vi "Station.Execution.vi"() -> ()   [LabVIEW 2015, in "Station.Execution.lvlib"]
uses:
  Station.Execution.lvlib
  Types/Main.StateVariables.ctl
  Types/Execute.UserEventRefs.ctl
  <vilib>/NI Veristand/Execution/Workspace/SystemStateRegEventRef.ctl
  <vilib>/NI Veristand/Execution/Workspace/Target State Info.ctl
  <vilib>/NI Veristand/Execution/Workspace/Target State.ctl
  <vilib>/NI Veristand/Execution/WaveformStreaming/Waveform Data Watcher Event Data (DBL).ctl
  <vilib>/NI Veristand/Execution/WaveformStreaming/WaveformStreamSpecification.ctl
  <vilib>/NI Veristand/Execution/Workspace/SystemStateEventRef.ctl
  <vilib>/NI Veristand/Execution/Workspace/WorkspaceAPI.ctl
  Types/UI.Tables.ctl
  Types/UI.Object.ctl
  Types/Waveforms.Info.ctl
  <vilib>/NI Veristand/Execution/WaveformStreaming/Registered Waveform Streams Data Event Refnum (DBL).ctl
  <vilib>/NI Veristand/Execution/WaveformStreaming/WaveformDataWatcherDBL.ctl
  <vilib>/NI Veristand/Execution/WaveformStreaming/WaveformStreamingAPI.ctl
  <vilib>/NI/AMC/Read Termination Message.vi
  <vilib>/NI/AMC/Update Message Routing Info.vi
  <vilib>/NI/AMC/Create Multiple Messages.vi
  <vilib>/NI/AMC/Create Single Message.vi
  <vilib>/NI/AMC/Globals.vi
  <vilib>/NI/AMC/Send Message.vi
  NationalInstruments.VeriStand.ClientAPI
  <vilib>/NI Veristand/Execution/Workspace/NI_VS Workspace ExecutionAPI.lvlib
  <vilib>/NI/AMC/AMC.lvlib
  <vilib>/NI Veristand/Execution/WaveformStreaming/NI_VS Waveform Streaming Interface.lvlib
panel:
  in  "Station.ID":string="DUT1"
  out "Station ID":string="Station 1"
  in  "NIVS.Gateway IP Address":string="localhost"
  in  "NIVS.Workspace Event":refnum<event-registration>
  in  "ToolTab":enum32{"Enable", "Disable"}(tab)
  in  "Back":bool
  in  "Next":bool
  in  "Pages":T1(tab)
  out "CAN.ODH":string[][](table)
  out "DAQ.ODH":string[][](table)
  out "CAN.IDL":string[][](table)
  out "DAQ.IDL":string[][](table)
  out "CAN.IDH":string[][](table)
  out "DAQ.IDH":string[][](table)
  out "CAN.OPH":string[][](table)
  out "DAQ.OPH":string[][](table)
  out "CAN.ODL":string[][](table)
  out "DAQ.ODL":string[][](table)
  out "CAN.Fault Status":string[][](table)
  out "CAN.LIN":string[][](table)
  in  "Waveform.Select":bool
  out "Waveform.Graph":waveform(dbl)[](graph)
  in  "Waveform.Groups":u8(ring) items=["", "All", "Eat", "Slow", "Test"]
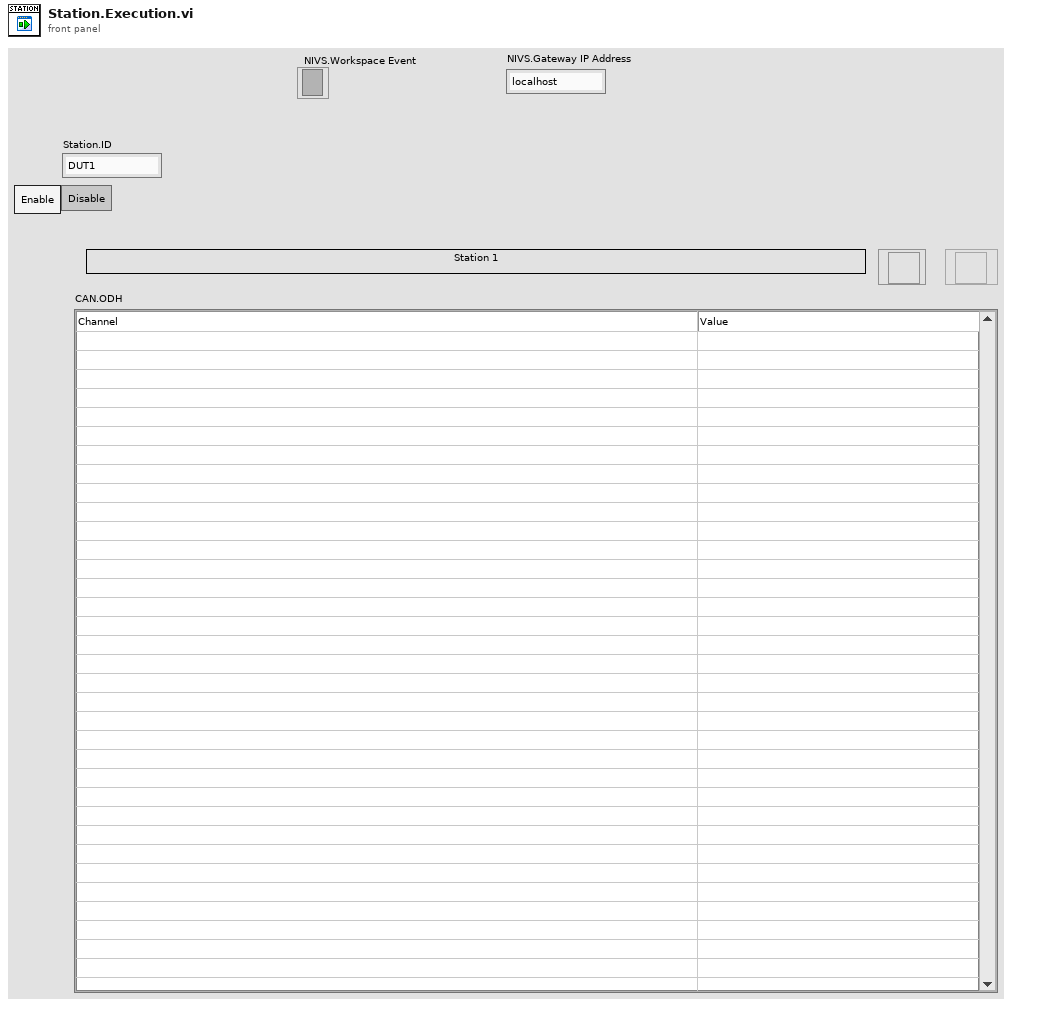
[diagram p1: front panel]
types:
  T1 = enum32{"CAN.ODH", "DAQ.ODH", "CAN.IDL", "DAQ.IDL", "CAN.IDH", "DAQ.IDH", "CAN.OPH", "DAQ.OPH", "CAN.ODL", "DAQ.ODL", "CAN.Fault Status", "CAN.LIN", "OSCOPE"}
  T2 = typedef "Station.Execution.lvlib/Main.StateVariables.ctl" = cluster{"NIVS.Deployed":bool, "NIVS.Events":T3, "NIVS.GatewayIPAddress":string, "NIVS.SystemDefinitionFile":path, "NIVS.SystemStateRefs":T5, "NIVS.WorkspaceManager":T6, "Station.ID":string, "UI.Back":refnum<vi>, "UI.Next":refnum<vi>, "UI.Pages":refnum<vi>, "UI.ToolTab":refnum<vi>, "Tables":T7, "VI.Ref":refnum<vi>, "NIVS.Open":bool, "Waveform.Groups":refnum<vi>, "Waveform.Select":refnum<vi>, "Waveform.Graph":refnum<vi>, "Waveforms.Info":T9[], "Waveforms":cluster{"Refs":T10[], "Event.Refs":T11, "Streaming.Ref":T13}, "Waveforms.Reset":bool}
  T3 = typedef "Station.Execution.lvlib/Execute.UserEventRefs.ctl" = cluster{"SystemChangeEvent":T4, "WorkspaceEvent":refnum<event-registration>, "WaveformEvent":refnum<event-registration>}
  T4 = typedef "NI_VS Workspace ExecutionAPI.lvlib/SystemStateRegEventRef.ctl" = refnum<event-registration>
  T5 = typedef "NI_VS Workspace ExecutionAPI.lvlib/SystemStateEventRef.ctl" = cluster{"CustDatRef":refnum<user-event>, "EvtRef":refnum<k27>, "Target State User Event":refnum<user-event>}
  T6 = typedef "NI_VS Workspace ExecutionAPI.lvlib/WorkspaceAPI.ctl" = refnum<k24>
  T7 = typedef "Station.Execution.lvlib/UI.Tables.ctl" = cluster{"CAN.Fault Status":T8, "CAN.IDH":T8, "CAN.IDL":T8, "CAN.LIN":T8, "CAN.ODH":T8, "CAN.ODL":T8, "CAN.OPH":T8, "DAQ.IDH":T8, "DAQ.IDL":T8, "DAQ.ODH":T8, "DAQ.ODL":T8, "DAQ.OPH":T8}
  T8 = typedef "Station.Execution.lvlib/UI.Object.ctl" = cluster{"Ref":refnum<vi>, "Paths":string[], "Names":string[]}
  T9 = typedef "Station.Execution.lvlib/Waveforms.Info.ctl" = cluster{"Name":string, "Path":string}
  T10 = typedef "NI_VS Waveform Streaming Interface.lvlib/WaveformStreamSpecification.ctl" = refnum<k24>
  T11 = typedef "NI_VS Waveform Streaming Interface.lvlib/Registered Waveform Streams Data Event Refnum (DBL).ctl" = cluster{"Callback Refnum":refnum<k27>, "Data Event":refnum<user-event>, "Event Refnum":refnum<event-registration>, "WaveformDataWatcherDBL":T12}
  T12 = typedef "NI_VS Waveform Streaming Interface.lvlib/WaveformDataWatcherDBL.ctl" = refnum<k24>
  T13 = typedef "NI_VS Waveform Streaming Interface.lvlib/WaveformStreamingAPI.ctl" = refnum<k24>
  T14 = typedef "AMC.lvlib/Message Queue.ctl" = refnum<queue>
  T15 = enum8{"Enabled", "Disabled", "Disabled and Grayed Out"}
  T16 = cluster{"Waveform.Refs":T10[], "WaveformStreaming.Event.Refs":T11, "WaveformStreaming.Ref":T13}
  T17 = typedef "AMC.lvlib/Message.ctl" = cluster{"name":string, "value":string, "attributes":T18, "receiver host":string, "receiver process":string, "source host":string, "source process":string, "priority message":bool, "acknowledge message":bool}
  T18 = typedef "Tools_KeyedArray.lvlib/KeyedArray.ctl" = cluster{"keys":string[], "values":string[]}
  T19 = cluster{"Refs":T10[], "Event.Refs":T11, "Streaming.Ref":T13}
  T20 = typedef "NI_VS Workspace ExecutionAPI.lvlib/SystemState.ctl" = u8
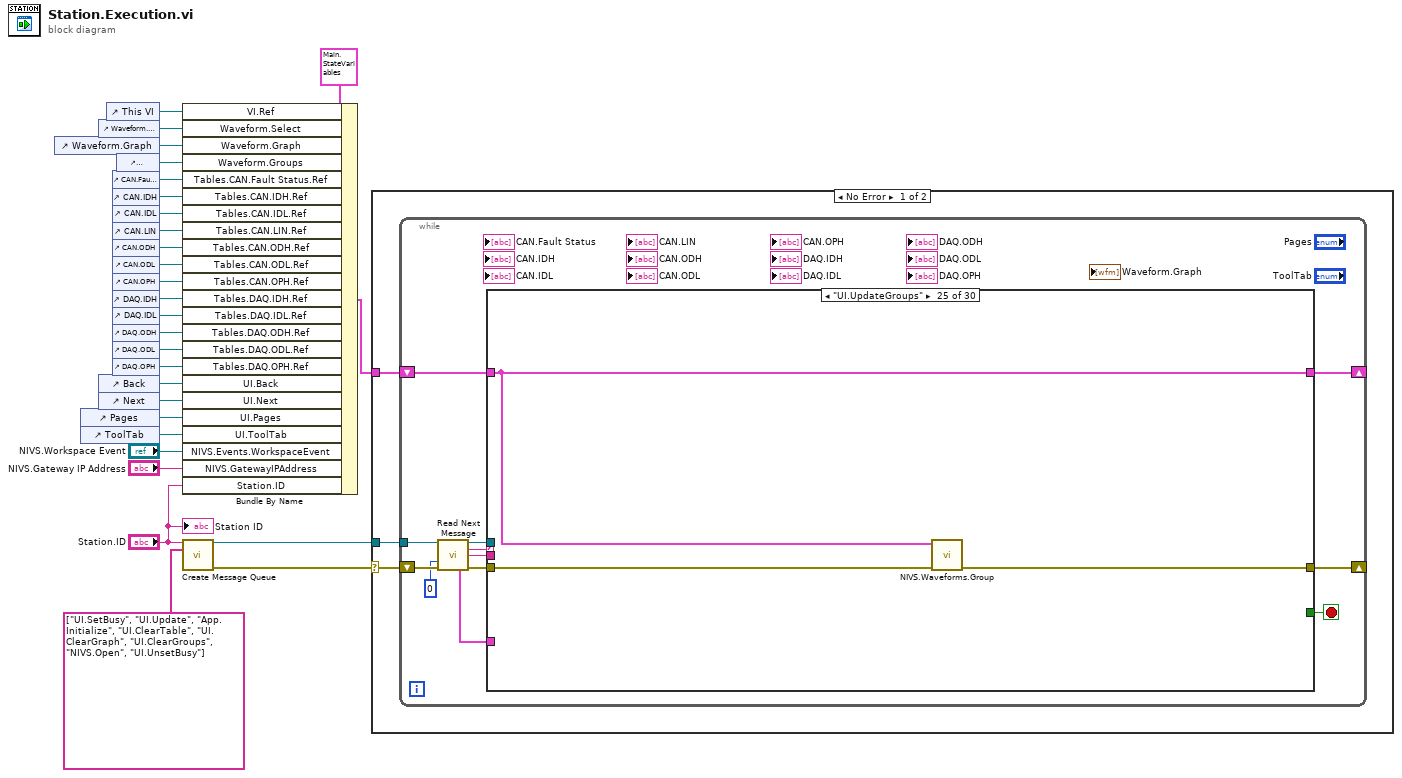
[diagram p0: block diagram]
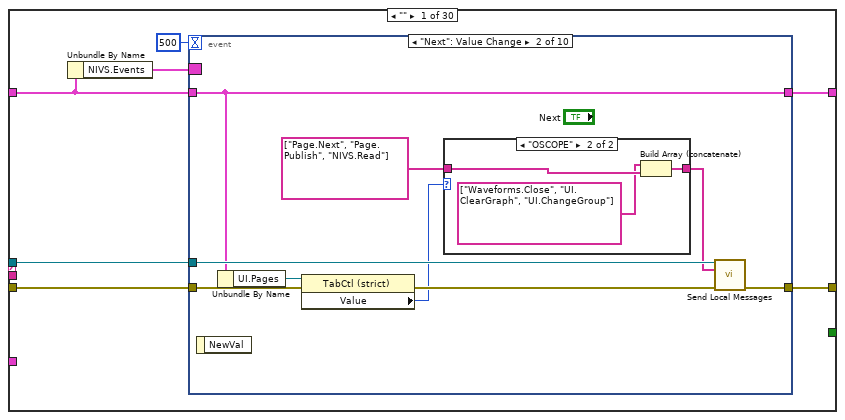
[diagram p2: hidden frame]
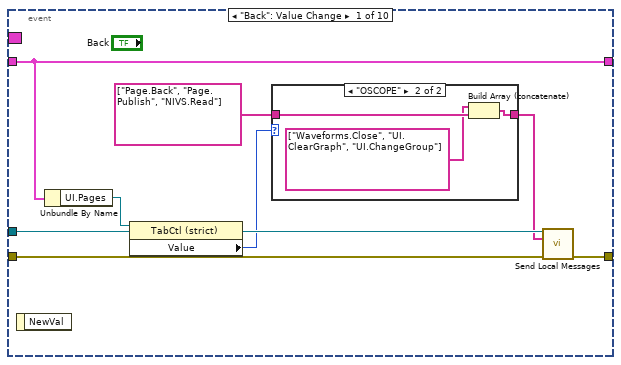
[diagram p3: hidden frame]
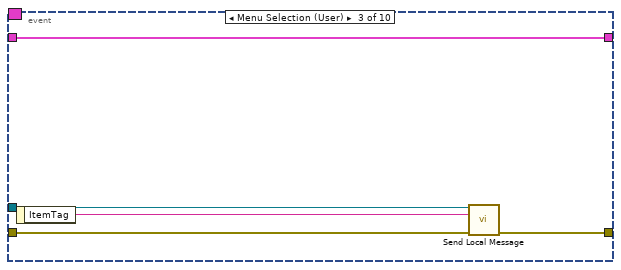
[diagram p6: hidden frame]
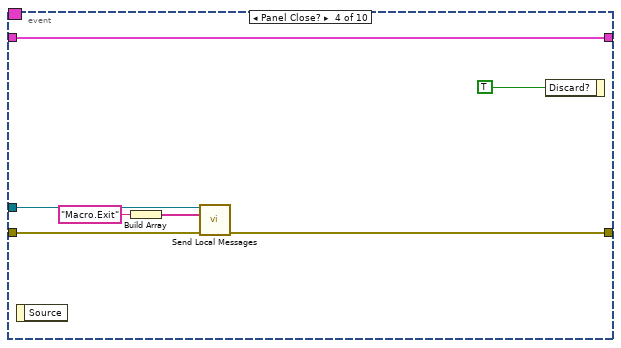
[diagram p7: hidden frame]
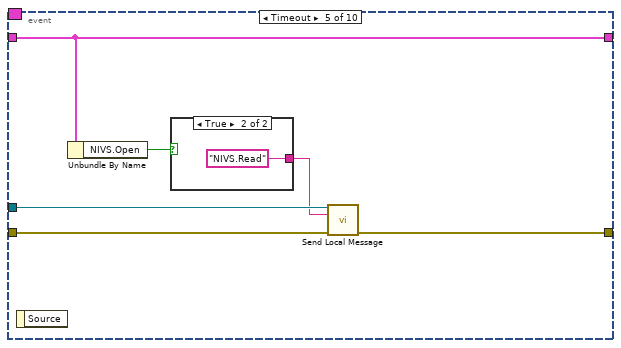
[diagram p8: hidden frame]
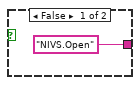
[diagram p9: hidden frame]
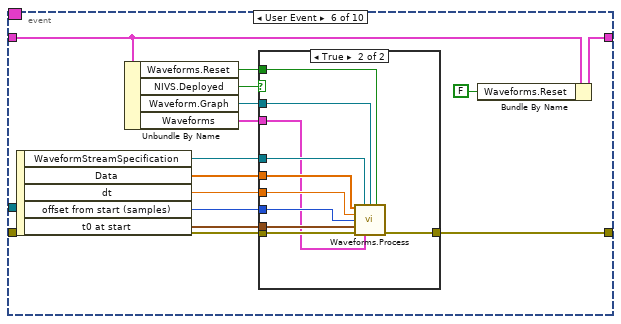
[diagram p10: hidden frame]
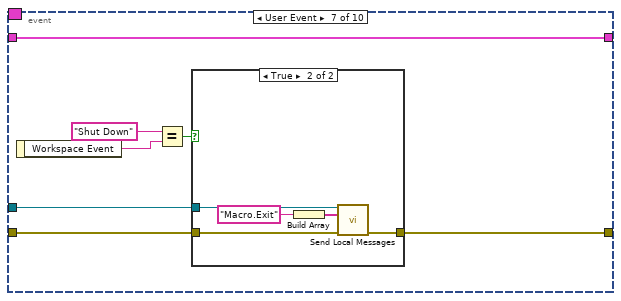
[diagram p12: hidden frame]
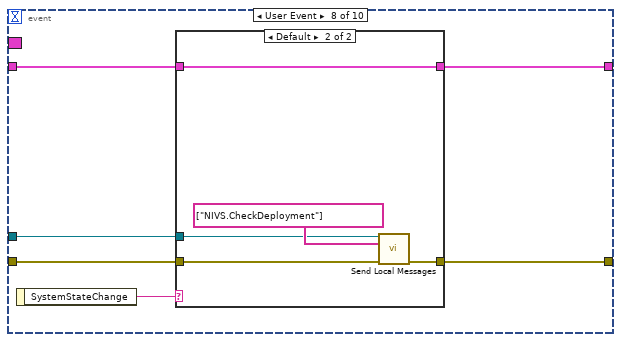
[diagram p14: hidden frame]
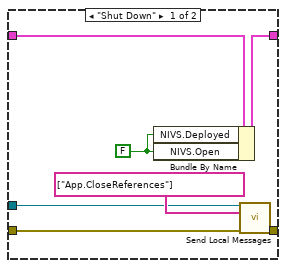
[diagram p15: hidden frame]
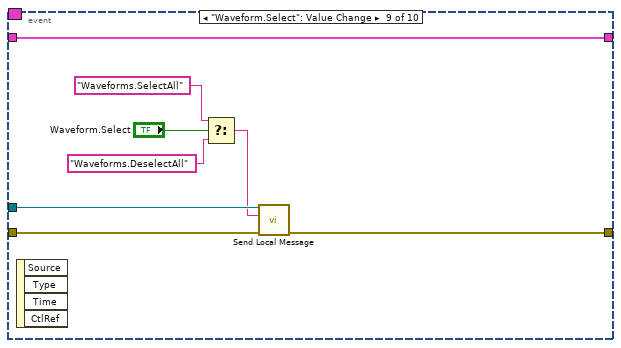
[diagram p16: hidden frame]
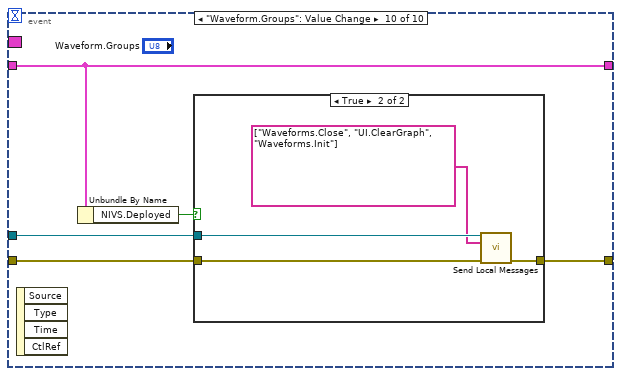
[diagram p17: hidden frame]
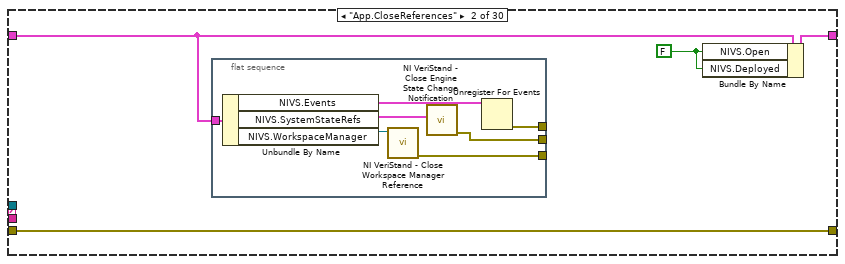
[diagram p19: hidden frame]
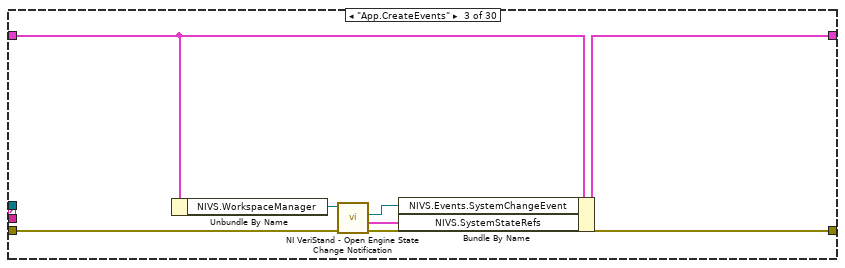
[diagram p20: hidden frame]
diagram:
  n1 = control-ref of="Waveform.Graph"() -> (w1:refnum<vi>)
  n2 = control-ref of="Pages"() -> (w5:refnum<vi>)
  n3 = control-ref of="ToolTab"() -> (w23:refnum<vi>)
  n4 = control-ref of="Waveform.Select"() -> (w2:refnum<vi>)
  n5 = control-ref of="Back"() -> (w21:refnum<vi>)
  n6 = control-ref of="Next"() -> (w22:refnum<vi>)
  n7 = control-ref of="This VI"() -> (w4:refnum<vi>)
  n8 = control-ref of="CAN.Fault Status"() -> (w16:refnum<vi>)
  n9 = control-ref of="CAN.IDH"() -> (w15:refnum<vi>)
  n10 = control-ref of="CAN.IDL"() -> (w14:refnum<vi>)
  n11 = control-ref of="CAN.LIN"() -> (w13:refnum<vi>)
  n12 = control-ref of="CAN.ODH"() -> (w12:refnum<vi>)
  n13 = control-ref of="CAN.ODL"() -> (w11:refnum<vi>)
  n14 = control-ref of="CAN.OPH"() -> (w10:refnum<vi>)
  n15 = control-ref of="DAQ.IDH"() -> (w9:refnum<vi>)
  n16 = control-ref of="DAQ.IDL"() -> (w8:refnum<vi>)
  n17 = control-ref of="DAQ.ODH"() -> (w17:refnum<vi>)
  n18 = control-ref of="DAQ.ODL"() -> (w18:refnum<vi>)
  n19 = control-ref of="DAQ.OPH"() -> (w19:refnum<vi>)
  n20 = control-ref of="Waveform.Groups"() -> (w3:refnum<vi>)
  n21 = Bundle By Name(cluster=T2 {"NIVS.Deployed"=FALSE, "NIVS.Events"={"SystemChangeEvent"=refnum, "WorkspaceEvent"=refnum, "WaveformEvent"=refnum}, "NIVS.GatewayIPAddress"="", "NIVS.SystemDefinitionFile"=path "", "NIVS.SystemStateRefs"={"CustDatRef"=refnum, "EvtRef"=refnum, "Target State User Event"=refnum}, "NIVS.WorkspaceManager"=refnum, "Station.ID"="", "UI.Back"=refnum, "UI.Next"=refnum, "UI.Pages"=refnum, "UI.ToolTab"=refnum, "Tables"={"CAN.Fault Status"={"Ref"=refnum, "Paths"=[], "Names"=[]}, "CAN.IDH"={"Ref"=refnum, "Paths"=[], "Names"=[]}, "CAN.IDL"={"Ref"=refnum, "Paths"=[], "Names"=[]}, "CAN.LIN"={"Ref"=refnum, "Paths"=[], "Names"=[]}, "CAN.ODH"={"Ref"=refnum, "Paths"=[], "Names"=[]}, "CAN.ODL"={"Ref"=refnum, "Paths"=[], "Names"=[]}, "CAN.OPH"={"Ref"=refnum, "Paths"=[], "Names"=[]}, "DAQ.IDH"={"Ref"=refnum, "Paths"=[], "Names"=[]}, "DAQ.IDL"={"Ref"=refnum, "Paths"=[], "Names"=[]}, "DAQ.ODH"={"Ref"=refnum, "Paths"=[], "Names"=[]}, "DAQ.ODL"={"Ref"=refnum, "Paths"=[], "Names"=[]}, "DAQ.OPH"={"Ref"=refnum, "Paths"=[], "Names"=[]}}, "VI.Ref"=refnum, "NIVS.Open"=FALSE, "Waveform.Groups"=refnum, "Waveform.Select"=refnum, "Waveform.Graph"=refnum, "Waveforms.Info"=[], "Waveforms"={"Refs"=[], "Event.Refs"={"Callback Refnum"=refnum, "Data Event"=refnum, "Event Refnum"=refnum, "WaveformDataWatcherDBL"=refnum}, "Streaming.Ref"=refnum}, "Waveforms.Reset"=FALSE} ("Cluster"), "VI.Ref"=w4, "Waveform.Select"=w2, "Waveform.Graph"=w1, "Waveform.Groups"=w3, "Tables.CAN.Fault Status.Ref"=w16, "Tables.CAN.IDH.Ref"=w15, "Tables.CAN.IDL.Ref"=w14, "Tables.CAN.LIN.Ref"=w13, "Tables.CAN.ODH.Ref"=w12, "Tables.CAN.ODL.Ref"=w11, "Tables.CAN.OPH.Ref"=w10, "Tables.DAQ.IDH.Ref"=w9, "Tables.DAQ.IDL.Ref"=w8, "Tables.DAQ.ODH.Ref"=w17, "Tables.DAQ.ODL.Ref"=w18, "Tables.DAQ.OPH.Ref"=w19, "UI.Back"=w21, "UI.Next"=w22, "UI.Pages"=w5, "UI.ToolTab"=w23, "NIVS.Events.WorkspaceEvent"="NIVS.Workspace Event", "NIVS.GatewayIPAddress"="NIVS.Gateway IP Address", "Station.ID"="Station.ID") -> (w28:T2)
  n22 = call <vilib>:"Create Message Queue.vi"("message queue name"="Station.ID", "initial message names"=string[] ["UI.SetBusy", "UI.Update", "App.Initialize", "UI.ClearTable", "UI.ClearGraph", "UI.ClearGroups", "NIVS.Open", "UI.UnsetBusy"]) -> ("message queue out"=w25:T14, "error out"=w6:errorcluster)  [unwired: 12 in]
  n23 = case shown="No Error" w6 {
    selector: w6 -> [w29 _]
    tunnel: w28 -> [w30 _]
    tunnel: w25 -> [w31 _]
    frame No Error {
      n24 = while {
        shift-right: [w42] -> _
        shift-left: w30 -> [w43]
        shift-right: [w32] -> _
        shift-left: w29 -> [w41]
        tunnel: w31 -> [w39]
        stop <- w40 stop-if-true
        n25 = call <vilib>:"Read Next Message.vi"("message queue in"=w39, "timeout (1 ms)"=0 ("Timeout"), "error in"=w41) -> ("message queue out"=w36:T14, "message name"=w35:string, "message value"=w34:string, "message"=w33:T17, "error out"=w37:errorcluster)  [unwired: 5 in, 3 out]
        n26 = case shown="\"UI.UpdateGroups\"" w35 {
          selector: w35 -> [_ _ _ _ _ _ _ _ _ _ _ _ _ _ _ _ _ w338 w344 _ _ _ _ _ _ _ _ _ _ _]
          tunnel: w43 -> [w46 w172 w181 w188 w193 w199 w214 w218 w237 w267 w271 w272 w293 w324 w328 w331 w333 w342 w347 w355 w358 w370 w376 w381 w384 w387 w396 w412 w436 w447]
          tunnel: [w50 w171 w182 w188 w193 w199 w214 w217 w236 w263 w271 w272 w293 w324 w328 w331 w332 w342 w347 w355 w358 w370 w376 w381 w384 w386 w395 w412 w436 w447] -> w42
          tunnel: [w47 w173 w184 w189 w194 w203 w212 w224 w238 w265 w269 w274 w292 w310 w325 w329 w334 w339 w343 w348 w356 w368 w373 w378 w382 w385 w397 w401 w425 w446] -> w32
          tunnel: w37 -> [w48 w173 w183 w190 w195 w202 w213 w219 w239 w268 w270 w273 w291 w310 w326 w330 w334 w339 w343 w349 w357 w363 w374 w379 w383 w390 w394 w404 w428 w446]
          tunnel: [_ _ _ TRUE _ _ _ _ _ _ _ _ _ _ _ _ _ _ _ _ _ _ _ _ _ _ _ _ _ _] -> w40
          tunnel: w36 -> [w44 _ _ w191 _ w200 w211 w223 w235 _ _ _ _ _ _ _ _ _ _ _ _ _ _ _ _ _ _ _ _ _]
          tunnel: w34 -> [_ _ _ _ _ _ _ _ _ _ _ _ _ _ w327 _ _ _ _ _ _ _ _ _ _ _ _ _ _ _]
          tunnel: w33 -> [_ _ _ _ _ _ _ _ _ _ _ _ _ _ _ _ _ _ _ _ _ _ _ _ _ _ _ _ _ _]
          frame "" {
            n27 = Unbundle By Name(w46) -> ("NIVS.Events"=w45:T3)
            n28 = event shown="[1] \"Next\": Value Change" {
              selector: w45 -> [_ _ _ _ _ _ _ _ _ _]
              dyn-events: _ -> [_ _ _ _ _ _ _ _ _ _]
              timeout: 500 -> [_ _ _ _ _ _ _ _ _ _]
              tunnel: [w52 w69 w76 w86 w89 w97 w125 w134 w159 w161] -> w50
              tunnel: w46 -> [w52 w69 w76 w86 w89 w98 w125 w135 w159 w161]
              tunnel: [w57 w71 w79 w83 w91 w108 w123 w136 w157 w163] -> w47
              tunnel: w48 -> [w58 w67 w80 w84 w92 w109 w124 w139 w158 w164]
              tunnel: w44 -> [w56 w70 w78 w82 w93 _ w122 w138 w156 w162]
              event "Back": Value Change {
                n29 = event-data() -> ()  [unwired: 1 in, 1 out]
                n30 = Unbundle By Name(w52) -> ("UI.Pages"=w51:refnum<vi>)
                n31 = property class="TabCtl (strict)"(reference=w51) -> ("Value"=w55:T1)  [unwired: 1 in, 2 out]
                n32 = case shown="\"OSCOPE\"" w55 {
                  tunnel: [w59 w61] -> w54
                  tunnel: string[] ["Page.Back", "Page.Publish", "NIVS.Read"] ("message names") -> [w59 w62]
                  frame Default {
                  }
                  frame "OSCOPE" {
                    n33 = Build Array (concatenate)(string[] ["Waveforms.Close", "UI.ClearGraph", "UI.ChangeGroup"], w62) -> (w61:string[])
                  }
                }
                n34 = call <vilib>:"Send Local Messages.vi"("message queue in"=w56, "message names"=w54, "error in"=w58) -> ("error out"=w57:errorcluster)  [unwired: 10 in, 2 out]
              }
              event "Next": Value Change {
                n35 = event-data() -> ()  [unwired: 1 in, 1 out]
                n36 = Unbundle By Name(w69) -> ("UI.Pages"=w68:refnum<vi>)
                n37 = property class="TabCtl (strict)"(reference=w68, error in=w67) -> (error out=w66:errorcluster, "Value"=w65:T1)  [unwired: 1 out]
                n38 = case shown="\"OSCOPE\"" w65 {
                  tunnel: [w72 w74] -> w63
                  tunnel: string[] ["Page.Next", "Page.Publish", "NIVS.Read"] ("message names") -> [w72 w75]
                  frame Default {
                  }
                  frame "OSCOPE" {
                    n39 = Build Array (concatenate)(string[] ["Waveforms.Close", "UI.ClearGraph", "UI.ChangeGroup"], w75) -> (w74:string[])
                  }
                }
                n40 = call <vilib>:"Send Local Messages.vi"("message queue in"=w70, "message names"=w63, "error in"=w66) -> ("error out"=w71:errorcluster)  [unwired: 10 in, 2 out]
              }
              event Menu Selection (User) {
                n41 = event-data() -> ("ItemTag"=w77:string)  [unwired: 1 in]
                n42 = call <vilib>:"Send Local Message.vi"("message queue in"=w78, "message name"=w77, "error in"=w80) -> ("error out"=w79:errorcluster)  [unwired: 10 in, 2 out]
              }
              event Panel Close? {
                n43 = event-data() -> ()  [unwired: 1 in, 1 out]
                n44 = Build Array("Macro.Exit") -> (w81:string[])
                n45 = call <vilib>:"Send Local Messages.vi"("message queue in"=w82, "message names"=w81, "error in"=w84) -> ("error out"=w83:errorcluster)  [unwired: 10 in, 2 out]
                n46 = event-data("Discard?"=TRUE) -> ()  [unwired: 1 in, 1 out]
              }
              event Timeout {
                n47 = event-data() -> ()  [unwired: 1 in, 1 out]
                n48 = Unbundle By Name(w89) -> ("NIVS.Open"=w88:bool)
                n49 = case shown="True" w88 {
                  tunnel: ["NIVS.Open" ("message name") "NIVS.Read" ("message name")] -> w90
                  frame False {
                  }
                  frame True {
                  }
                }
                n50 = call <vilib>:"Send Local Message.vi"("message queue in"=w93, "message name"=w90, "error in"=w92) -> ("error out"=w91:errorcluster)  [unwired: 10 in, 2 out]
              }
              event User Event {
                n51 = event-data() -> ("WaveformStreamSpecification"=w107:T10, "Data"=w105:dbl[], "dt"=w104:dbl, "offset from start (samples)"=w103:u64, "t0 at start"=w102:timestamp)  [unwired: 1 in]
                n52 = Unbundle By Name(w98) -> ("Waveforms.Reset"=w99:bool, "NIVS.Deployed"=w100:bool, "Waveform.Graph"=w106:refnum<vi>, "Waveforms"=w101:T19)
                n53 = case shown="True" w100 {
                  tunnel: w109 -> [w110 w120]
                  tunnel: [w110 w119] -> w108
                  tunnel: w107 -> [_ w118]
                  tunnel: w106 -> [_ w117]
                  tunnel: w105 -> [_ w116]
                  tunnel: w104 -> [_ w115]
                  tunnel: w103 -> [_ w114]
                  tunnel: w102 -> [_ w113]
                  tunnel: w101 -> [_ w112]
                  tunnel: w99 -> [_ w111]
                  frame False {
                  }
                  frame True {
                    n54 = call "Waveforms.Process.vi"("Data"=w116, "Waveform.Ref"=w118, "WaveformGraph.Ref"=w117, "Reset?"=w111, "dt"=w115, "offset from start (samples)"=w114, "t0 at start"=w113, "error in (no error)"=w120, "Waveforms"=w112) -> ("error out"=w119:errorcluster)  [unwired: 6 in]
                  }
                }
                n55 = Bundle By Name(cluster=w98, "Waveforms.Reset"=FALSE) -> (w97:T2)
              }
              event User Event {
                n56 = event-data() -> ("Workspace Event"=w121:string)  [unwired: 1 in]
                n57 = Equal?(x="Shut Down" ("y"), y=w121) -> (x = y?=w126:bool)
                n58 = case shown="True" w126 {
                  tunnel: w124 -> [w128 w133]
                  tunnel: [w128 w132] -> w123
                  tunnel: w122 -> [_ w131]
                  frame False {
                  }
                  frame True {
                    n59 = Build Array("Macro.Exit" ("y")) -> (w130:string[])
                    n60 = call <vilib>:"Send Local Messages.vi"("message queue in"=w131, "message names"=w130, "error in"=w133) -> ("error out"=w132:errorcluster)  [unwired: 10 in, 2 out]
                  }
                }
              }
              event User Event {
                n61 = event-data() -> ("SystemStateChange"=w137:string)  [unwired: 1 in]
                n62 = case shown="Default" w137 {
                  tunnel: w139 -> [w145 w150]
                  tunnel: w138 -> [w144 w149]
                  tunnel: [w143 w148] -> w136
                  tunnel: w135 -> [w142 w147]
                  tunnel: [w141 w147] -> w134
                  frame "Shut Down" {
                    w140 = FALSE ("NIVS.Open")
                    n63 = Bundle By Name(cluster=w142, "NIVS.Deployed"=w140, "NIVS.Open"=w140) -> (w141:T2)
                    n64 = call <vilib>:"Send Local Messages.vi"("message queue in"=w144, "message names"=string[] ["App.CloseReferences"], "error in"=w145) -> ("error out"=w143:errorcluster)  [unwired: 10 in, 2 out]
                  }
                  frame Default {
                    n65 = call <vilib>:"Send Local Messages.vi"("message queue in"=w149, "message names"=string[] ["NIVS.CheckDeployment"], "error in"=w150) -> ("error out"=w148:errorcluster)  [unwired: 10 in, 2 out]
                  }
                }
              }
              event "Waveform.Select": Value Change {
                n66 = event-data() -> ()  [unwired: 1 in, 4 out]
                n67 = Select(t="Waveforms.SelectAll", s="Waveform.Select", f="Waveforms.DeselectAll") -> (s? t:f=w152:string)
                n68 = call <vilib>:"Send Local Message.vi"("message queue in"=w156, "message name"=w152, "error in"=w158) -> ("error out"=w157:errorcluster)  [unwired: 10 in, 2 out]
              }
              event "Waveform.Groups": Value Change {
                n69 = event-data() -> ()  [unwired: 1 in, 4 out]
                n70 = Unbundle By Name(w161) -> ("NIVS.Deployed"=w160:bool)
                n71 = case shown="True" w160 {
                  tunnel: w164 -> [w165 w169]
                  tunnel: [w165 w168] -> w163
                  tunnel: w162 -> [_ w167]
                  frame False {
                  }
                  frame True {
                    n72 = call <vilib>:"Send Local Messages.vi"("message queue in"=w167, "message names"=string[] ["Waveforms.Close", "UI.ClearGraph", "Waveforms.Init"], "error in"=w169) -> ("error out"=w168:errorcluster)  [unwired: 10 in, 2 out]
                  }
                }
              }
            }
          }
          frame "App.CloseReferences" {
            w170 = FALSE ("NIVS.Open")
            n73 = flat-sequence {
              tunnel: w172 -> [w177]
              tunnel: [w176] -> _
              tunnel: [w175] -> _
              tunnel: [w174] -> _
              frame #0 {
                n74 = Unbundle By Name(w177) -> ("NIVS.Events"=w178:T3, "NIVS.SystemStateRefs"=w180:T5, "NIVS.WorkspaceManager"=w179:T6)
                n75 = call <vilib>:"NI VeriStand - Close Workspace Manager Reference.vi"("WorkspaceManager"=w179) -> ("error out"=w174:errorcluster)  [unwired: 10 in]
                n76 = call <vilib>:"NI VeriStand - Close Engine State Change Notification.vi"("SystemStateRefs"=w180) -> ("error out"=w175:errorcluster)  [unwired: 10 in]
                n77 = Unregister For Events(event registration refnum=w178) -> (error out=w176:errorcluster)  [unwired: 1 in]
              }
            }
            n78 = Bundle By Name(cluster=w172, "NIVS.Open"=w170, "NIVS.Deployed"=w170) -> (w171:T2)
          }
          frame "App.CreateEvents" {
            n79 = Unbundle By Name(w181) -> ("NIVS.WorkspaceManager"=w185:T6)
            n80 = call <vilib>:"NI VeriStand - Open Engine State Change Notification.vi"("error in (no error)"=w183, "WorkspaceManager in"=w185) -> ("error out"=w184:errorcluster, "SystemStateRefs"=w187:T5, "SystemChangeEventRef"=w186:T4)  [unwired: 6 in, 1 out]
            n81 = Bundle By Name(cluster=w181, "NIVS.Events.SystemChangeEvent"=w186, "NIVS.SystemStateRefs"=w187) -> (w182:T2)
          }
          frame "App.Exit" {
            n82 = call <vilib>:"Destroy Message Queue.vi"("message queue in"=w191, "error in"=w190) -> ("error out"=w189:errorcluster)  [unwired: 11 in, 2 out]
          }
          frame "App.Initialize" {
            n83 = call "Execute.Initialize.vi"("error in (no error)"=w195, "State Variables"=w193) -> ("error out"=w194:errorcluster)  [unwired: 9 in]
          }
          frame "Error" {
            n84 = for {
              shift-right: [w208] -> w197
              shift-left: w202 -> [w209]
              tunnel: i32[] [-307652, -307654] -> [w207] mode=indexing
              n85 = call <vilib>:"Clear Errors.vi"("error in (no error)"=w209, "specific error code to clear (0: all)"=w207) -> ("error out"=w208:errorcluster)  [unwired: 4 in, 1 out]
            }
            n86 = case shown="Error" w197 {
              selector: w197 -> [w204 w205]
              tunnel: [w204 w206] -> w198
              frame No Error {
              }
              frame Error {
                n87 = call <vilib>:"Clear Errors.vi"("error in (no error)"=w205) -> ("error out"=w206:errorcluster)  [unwired: 5 in, 1 out]
                n88 = call "Error.Display.vi"("error in (no error)"=w205) -> ()  [unwired: 11 in]
              }
            }
            n89 = call <vilib>:"Send Local Messages.vi"("message queue in"=w200, "message names"=string[] ["UI.SetBusy", "UI.Update", "App.CloseReferences", "App.Initialize", "UI.ClearTable", "NIVS.Open", "UI.UnsetBusy"], "error in"=w198) -> ("error out"=w203:errorcluster)  [unwired: 10 in, 2 out]
          }
          frame "Macro.Exit" {
            n90 = call <vilib>:"Send Local Messages.vi"("message queue in"=w211, "message names"=string[] ["Waveforms.Close", "App.CloseReferences", "UI.Close", "App.Exit"], "error in"=w213) -> ("error out"=w212:errorcluster)  [unwired: 10 in, 2 out]
          }
          frame "NIVS.CheckDeployment" {
            n91 = Unbundle By Name(w218) -> ("NIVS.WorkspaceManager"=w221:T6)
            n92 = call <vilib>:"NI VeriStand - Get System State.vi"("error in (no error)"=w219, "WorkspaceManager in"=w221) -> ("error out"=w215:errorcluster, "System State"=w222:T20, "System Definition File"=w220:path)  [unwired: 5 in, 2 out]
            n93 = case shown="0, Default" w222 {
              tunnel: w218 -> [w229 w234]
              tunnel: [w228 w232] -> w217
              tunnel: w220 -> [_ w231]
              tunnel: [string[] ["Waveforms.Close", "UI.Update", "UI.ClearTable", "UI.ClearGraph", "UI.ClearGroups", "NIVS.GetChannels"] string[] ["UI.Update", "NIVS.GetChannels", "UI.UpdateGroups"]] -> w216
              frame 0, Default {
                # "Not connected"
                n94 = Bundle By Name(cluster=w229, "NIVS.Deployed"=FALSE ("Connected"), "NIVS.SystemDefinitionFile"=path "") -> (w228:T2)
              }
              frame 1 {
                # "Connected"
                n95 = Bundle By Name(cluster=w234, "NIVS.Deployed"=TRUE ("Connected"), "NIVS.SystemDefinitionFile"=w231) -> (w232:T2)
              }
            }
            n96 = call <vilib>:"Send Local Messages.vi"("message queue in"=w223, "message names"=w216, "error in"=w215) -> ("error out"=w224:errorcluster)  [unwired: 10 in, 2 out]
          }
          frame "NIVS.Open" {
            n97 = Unbundle By Name(w237) -> ("NIVS.GatewayIPAddress"=w240:string)
            n98 = case shown="No Error" w239 {
              selector: w239 -> [w243 w261]
              tunnel: w240 -> [w248 _]
              tunnel: [w242 w261] -> w238
              tunnel: w237 -> [w246 w262]
              tunnel: [w244 w262] -> w236
              tunnel: w235 -> [w241 _]
              frame No Error {
                n99 = call <vilib>:"NI VeriStand - Open Workspace Manager Reference.vi"("Gateway IP Address (\"\": localhost)"=w248) -> ("error out"=w247:errorcluster, "WorkspaceManager"=w245:T6)  [unwired: 9 in]
                n100 = case shown="No Error" w247 {
                  tunnel: w246 -> [w256 w259]
                  tunnel: w245 -> [w255 _]
                  tunnel: [w253 w258] -> w244
                  tunnel: w243 -> [w252 w260]
                  tunnel: [w251 w260] -> w242
                  tunnel: w241 -> [w250 _]
                  frame No Error {
                    n101 = Bundle By Name(cluster=w256, "NIVS.Open"=TRUE, "NIVS.WorkspaceManager"=w255) -> (w253:T2)
                    n102 = call <vilib>:"Send Local Messages.vi"("message queue in"=w250, "message names"=string[] ["App.CreateEvents", "NIVS.CheckDeployment"], "error in"=w252) -> ("error out"=w251:errorcluster)  [unwired: 10 in, 2 out]
                  }
                  frame Error {
                    n103 = Bundle By Name(cluster=w259, "NIVS.Open"=FALSE) -> (w258:T2)
                  }
                }
              }
              frame Error {
              }
            }
          }
          frame "NIVS.GetChannels" {
            n104 = call "NIVS.FilterChannels.vi"("error in (no error)"=w268, "Cluster in"=w267) -> ("error out"=w266:errorcluster, "Cluster out"=w264:T2)  [unwired: 8 in]
            n105 = call "NIVS.FilterWaveforms.vi"("error in (no error)"=w266, "Cluster in"=w264) -> ("error out"=w265:errorcluster, "Cluster out"=w263:T2)  [unwired: 8 in]
          }
          frame "NIVS.Read" {
            n106 = call "NIVS.Channels.Read.vi"("error in (no error)"=w270, "State Variables"=w271) -> ("error out"=w269:errorcluster)  [unwired: 9 in]
          }
          frame "Page.Back" {
            n107 = Unbundle By Name(w272) -> ("UI.Next"=w276:refnum<vi>, "UI.Back"=w283:refnum<vi>, "UI.Pages"=w288:refnum<vi>)
            n108 = property class="TabCtl (strict)"(reference=w288, error in=w273) -> (reference out=w286:refnum<vi>, error out=w285:errorcluster, "Value"=w287:T1)
            n109 = Decrement(x=w287) -> (x-1=w282:T1)
            n110 = Equal To 0?(x=w282) -> (x = 0?=w281:bool)
            n111 = property class="TabCtl (strict)"(reference=w286, error in=w285, "Value"=w282) -> (error out=w284:errorcluster)  [unwired: 1 out]
            n112 = Select(t=T15."Disabled and Grayed Out" ("Disabled"), s=w281, f=T15."Enabled") -> (s? t:f=w278:T15)
            n113 = property class="Bool"(reference=w283, error in=w284, "DisabledEnum"=w278) -> (error out=w277:errorcluster)  [unwired: 1 out]
            n114 = property class="Bool"(reference=w276, error in=w277, "DisabledEnum"=T15."Enabled" ("Disabled")) -> (error out=w274:errorcluster)  [unwired: 1 out]
          }
          frame "Page.Next" {
            n115 = Unbundle By Name(w293) -> ("UI.Back"=w309:refnum<vi>, "UI.Next"=w308:refnum<vi>, "UI.Pages"=w307:refnum<vi>)
            n116 = property class="TabCtl (strict)"(reference=w307, error in=w291) -> (reference out=w295:refnum<vi>, error out=w296:errorcluster, "Value"=w294:T1, "Pages"=w290:refnum<vi>[])
            n117 = To Unsigned Byte Integer(number=w294) -> (unsigned 8bit integer=w306:u8)
            n118 = Array Size(array=w290) -> (size(s)=w289:i32)
            n119 = Increment(x=w306) -> (x+1=w297:u8)
            n120 = Increment(x=w297) -> (x+1=w298:u8)
            n121 = property class="TabCtl (strict)"(reference=w295, error in=w296, "Value"=w297) -> (error out=w299:errorcluster)  [unwired: 1 out]
            n122 = Greater Or Equal?(x=w298, y=w289) -> (x >= y?=w304:bool)
            n123 = Select(t=T15."Disabled and Grayed Out" ("Disabled"), s=w304, f=T15."Enabled") -> (s? t:f=w305:T15)
            n124 = property class="Bool"(reference=w308, error in=w299, "DisabledEnum"=w305) -> (error out=w300:errorcluster)  [unwired: 1 out]
            n125 = property class="Bool"(reference=w309, error in=w300, "DisabledEnum"=T15."Enabled" ("Disabled")) -> (error out=w292:errorcluster)  [unwired: 1 out]
          }
          frame "Page.Publish" {
            n126 = Unbundle By Name(w324) -> ("Station.ID"=w318:string, "UI.Pages"=w323:refnum<vi>)
            n127 = property class="TabCtl (strict)"(reference=w323, error in=w310) -> (error out=w319:errorcluster, "Value"=w321:T1, "Pages"=w322:refnum<vi>[])  [unwired: 1 out]
            n128 = Index Array(array=w322, index=w321) -> (element=w320:refnum<vi>)
            n129 = property class="Page"(reference=w320, error in=w319) -> (error out=w314:errorcluster, "PageLabel"=w317:string)  [unwired: 1 out]
            n130 = Concatenate Strings(w318, "\\" ("string"), w317) -> (w315:string)
            n131 = call <vilib>:"Send Local Message.vi"("receiver process (\"\" - local)"="MainExecutionTool" ("string"), "message name"="Page.Published" ("string"), "message value"=w315, "error in"=w314) -> ("error out"=w311:errorcluster)  [unwired: 9 in, 2 out]
            n132 = call <vilib>:"Clear Errors.vi"("error in (no error)"=w311) -> ()  [unwired: 5 in, 2 out]
          }
          frame "Page.Set" {
            n133 = call "Page.Set.vi"("error in (no error)"=w326, "message value"=w327, "Cluster"=w328) -> ("error out"=w325:errorcluster)  [unwired: 8 in]
          }
          frame "UI.Open" {
            n134 = invoke class="VI" method="FP.Open"(error in=w330) -> (error out=w329:errorcluster)  [unwired: 4 in, 4 out]
          }
          frame "UI.Close" {
            n135 = flat-sequence {
              tunnel: [w336] -> w332
              tunnel: w333 -> [w336]
              tunnel: [w335] -> _
              frame #0 {
                n136 = invoke class="VI" method="FP.Close"() -> (error out=w335:errorcluster)  [unwired: 3 in, 2 out]
                n137 = Wait (ms)(milliseconds to wait=u32 500) -> ()  [unwired: 1 out]
              }
            }
          }
          frame "UI.SetBusy" {
            n138 = call <vilib>:"Send Local Message.vi"("receiver process (\"\" - local)"="MainExecutionTool" ("string"), "message name"=w338, "error in"=w339) -> ("error out"=w340:errorcluster)  [unwired: 10 in, 2 out]
            n139 = call <vilib>:"Clear Errors.vi"("error in (no error)"=w340) -> ()  [unwired: 5 in, 2 out]
            n140 = call <vilib>:"Set Busy.vi"() -> ()  [unwired: 10 in, 2 out]
          }
          frame "UI.UnsetBusy" {
            n141 = call <vilib>:"Send Local Message.vi"("receiver process (\"\" - local)"="MainExecutionTool" ("string"), "message name"=w344, "error in"=w343) -> ("error out"=w345:errorcluster)  [unwired: 10 in, 2 out]
            n142 = call <vilib>:"Clear Errors.vi"("error in (no error)"=w345) -> ()  [unwired: 5 in, 2 out]
            n143 = call <vilib>:"Unset Busy.vi"() -> ()  [unwired: 11 in, 1 out]
          }
          frame "UI.Update" {
            n144 = Unbundle By Name(w355) -> ("UI.ToolTab"=w354:refnum<vi>, "NIVS.Deployed"=w353:bool)
            n145 = Select(t=enum32{"Enable", "Disable"}."Enable" ("Value"), s=w353, f=enum32{"Enable", "Disable"}."Disable") -> (s? t:f=w350:enum32{"Enable", "Disable"})
            n146 = property class="TabCtl (strict)"(reference=w354, error in=w349, "Value"=w350) -> (error out=w348:errorcluster)  [unwired: 1 out]
          }
          frame "UI.ClearTable" {
            n147 = call "Table.Clear.vi"("error in (no error)"=w357, "State Variables"=w358) -> ("error out"=w356:errorcluster)  [unwired: 9 in]
          }
          frame "UI.ClearGraph" {
            n148 = Unbundle By Name(w370) -> ("Waveform.Graph"=w365:refnum<vi>)
            n149 = invoke class="WFGraph (strict)" method="Reinit To Default"(reference=w365, error in=w363) -> (reference out=w364:refnum<vi>, error out=w362:errorcluster)  [unwired: 1 in, 1 out]
            n150 = property class="WFGraph (strict)"(reference=w364, error in=w362, "Value"=waveform(dbl)[] [{"t0"=timestamp(0 s since 1904-01-01), "dt"=1.0, "Y"=[]}], "LegNumRows"=u32 1 ("Legend:Number of Rows"), "Active Plot"=u32 0, "Plot.Plot Name"="Plot 0", "LegScrollPos"=u32 0 ("Legend:Scroll Position"), "LegScrollVis"=FALSE ("Legend:Scrollbar Visible")) -> (error out=w368:errorcluster)  [unwired: 1 out]
          }
          frame "UI.ClearGroups" {
            n151 = Unbundle By Name(w376) -> ("Waveform.Groups"=w375:refnum<vi>)
            n152 = property class="Ring (strict)"(reference=w375, error in=w374, "Strings []"=string[] [], "Value"=u8 0) -> (error out=w373:errorcluster)  [unwired: 1 out]
          }
          frame "UI.ChangeGroup" {
            n153 = Unbundle By Name(w381) -> ("Waveform.Groups"=w380:refnum<vi>)
            n154 = property class="Ring (strict)"(reference=w380, error in=w379, "Value"=u8 0) -> (error out=w378:errorcluster)  [unwired: 1 out]
          }
          frame "UI.UpdateGroups" {
            n155 = call "NIVS.Waveforms.Group.vi"("error in (no error)"=w383, "Cluster"=w384) -> ("error out"=w382:errorcluster)  [unwired: 9 in]
          }
          frame "Waveforms.Close" {
            n156 = Unbundle By Name(w387) -> ("Waveforms"=w389:T19)
            n157 = flat-sequence {
              tunnel: w390 -> [w391]
              tunnel: [w393] -> _
              tunnel: w389 -> [w392]
              tunnel: [w391] -> w385
              frame #0 {
                n158 = call "Waveforms.Close.vi"("error in (no error)"=w391, "Waveforms"=w392) -> ("error out"=w393:errorcluster)  [unwired: 9 in]
              }
            }
            n159 = Bundle By Name(cluster=w387, "Waveforms"=T16 {"Waveform.Refs"=[], "WaveformStreaming.Event.Refs"={"Callback Refnum"=refnum, "Data Event"=refnum, "Event Refnum"=refnum, "WaveformDataWatcherDBL"=refnum}, "WaveformStreaming.Ref"=refnum} ("Waveforms.Refs")) -> (w386:T2)
          }
          frame "Waveforms.Init" {
            n160 = call "Waveforms.Start.vi"("error in (no error)"=w394, "Cluster in"=w396) -> ("error out"=w397:errorcluster, "Cluster out"=w395:T2)  [unwired: 8 in]
          }
          frame "Waveforms.SelectAll" {
            n161 = Unbundle By Name(w412) -> ("Waveform.Graph"=w411:refnum<vi>, "VI.Ref"=w407:refnum<vi>)
            n162 = property class="VI"(reference=w407, error in=w404) -> (error out=w405:errorcluster, "Panel"=w406:refnum<vi>)  [unwired: 1 out]
            n163 = property class="Pnl"(reference=w406, error in=w405, "DeferPanUpdts"=TRUE ("Defer Panel Updates")) -> (reference out=w399:refnum<vi>, error out=w403:errorcluster)
            n164 = property class="WFGraph (strict)"(reference=w411, error in=w403) -> (reference out=w409:refnum<vi>, error out=w408:errorcluster, "LegNumRows"=w410:u32)
            n165 = for {
              N: w410 -> [_]
              tunnel: w409 -> [w421]
              shift-right: [w417] -> w400
              shift-left: w408 -> [w420]
              i -> [w419]
              n166 = property class="WFGraph (strict)"(reference=w421, error in=w420, "Active Plot"=w419, "Plot.Visible?"=TRUE ("Legend:Visible")) -> (error out=w417:errorcluster)  [unwired: 1 out]
            }
            n167 = flat-sequence {
              tunnel: [w416] -> w401
              tunnel: w400 -> [w416]
              tunnel: w399 -> [w415]
              tunnel: FALSE ("Defer Panel Updates") -> [w414]
              tunnel: [w413] -> _
              frame #0 {
                n168 = property class="Pnl"(reference=w415, "DeferPanUpdts"=w414) -> (error out=w413:errorcluster)  [unwired: 1 in, 1 out]
              }
            }
          }
          frame "Waveforms.DeselectAll" {
            n169 = Unbundle By Name(w436) -> ("Waveform.Graph"=w435:refnum<vi>, "VI.Ref"=w431:refnum<vi>)
            n170 = property class="VI"(reference=w431, error in=w428) -> (error out=w429:errorcluster, "Panel"=w430:refnum<vi>)  [unwired: 1 out]
            n171 = property class="Pnl"(reference=w430, error in=w429, "DeferPanUpdts"=TRUE ("Defer Panel Updates")) -> (reference out=w423:refnum<vi>, error out=w427:errorcluster)
            n172 = property class="WFGraph (strict)"(reference=w435, error in=w427) -> (reference out=w433:refnum<vi>, error out=w432:errorcluster, "LegNumRows"=w434:u32)
            n173 = for {
              N: w434 -> [_]
              tunnel: w433 -> [w445]
              shift-right: [w441] -> w424
              shift-left: w432 -> [w444]
              i -> [w443]
              n174 = property class="WFGraph (strict)"(reference=w445, error in=w444, "Active Plot"=w443, "Plot.Visible?"=FALSE ("Legend:Visible")) -> (error out=w441:errorcluster)  [unwired: 1 out]
            }
            n175 = flat-sequence {
              tunnel: [w440] -> w425
              tunnel: w424 -> [w440]
              tunnel: w423 -> [w439]
              tunnel: FALSE ("Defer Panel Updates") -> [w438]
              tunnel: [w437] -> _
              frame #0 {
                n176 = property class="Pnl"(reference=w439, "DeferPanUpdts"=w438) -> (error out=w437:errorcluster)  [unwired: 1 in, 1 out]
              }
            }
          }
          frame Default {
          }
        }
      }
    }
    frame Error {
      n177 = disable-structure shown="Enabled" {
        frame Enabled {
          n178 = invoke class="VI" method="FP.Close"() -> ()  [unwired: 3 in, 3 out]
        }
        frame Disabled {
        }
      }
    }
  }
  "Station ID" <- "Station.ID"
